vi "CloseHardware.vi"(8 "error in (no error)":errorcluster, 11 "ThorLabsCsCamera in":refnum<class "ThorLabsCsCamera.lvclass">) -> (0 "error out":errorcluster, 3 "ThorLabsCsCamera out":refnum<class "ThorLabsCsCamera.lvclass">)   [LabVIEW 2020, in "ThorLabsCsCamera.lvclass"]
uses:
  ThorLabsCsCamera.lvclass
  ThorLabsCsCamera.lvclass/ThorLabsCsCamera.ctl
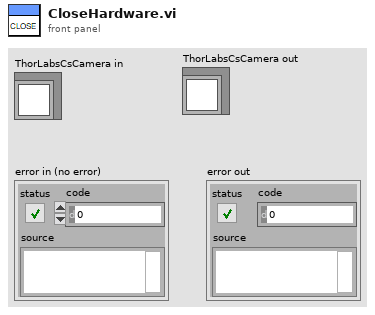
[diagram p1: front panel]
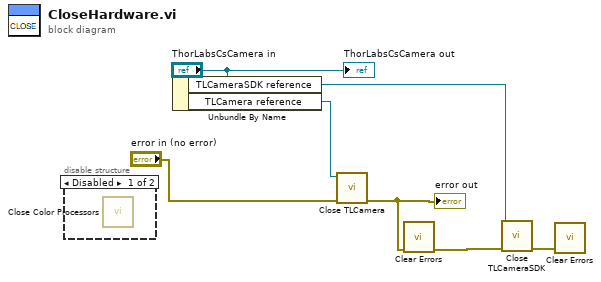
[diagram p0: block diagram]
diagram:
  n1 = disable-structure shown="Disabled" {
    frame Disabled {
      n2 = call "Close Color Processors.vi"() -> ()  [unwired: 11 in, 1 out]
    }
    frame Enabled {
    }
  }
  n3 = Unbundle By Name("ThorLabsCsCamera in") -> ("TLCameraSDK reference"=w2:refnum<k24>, "TLCamera reference"=w5:refnum<k24>)
  n4 = call "Close TLCamera.vi"("error in (no error)"="error in (no error)", "TLCamera reference"=w5) -> ("error out"=w3:errorcluster)  [unwired: 9 in]
  "error out" <- w3
  n5 = call "Clear Errors.vi"("error in (no error)"=w3) -> ("error out"=w4:errorcluster)  [unwired: 5 in, 1 out]
  n6 = call "Close TLCameraSDK.vi"("error in (no error)"=w4, "TLCameraSDK reference"=w2) -> ("error out"=w1:errorcluster)  [unwired: 9 in]
  n7 = call "Clear Errors.vi"("error in (no error)"=w1) -> ()  [unwired: 5 in, 2 out]
  "ThorLabsCsCamera out" <- "ThorLabsCsCamera in"
